vi "2D In Bounds Check.vi"(10 "Bounds":T2, 11 "Point in":cluster{"H":T1, "V":T1}) -> (2 "In Bounds?":bool, 3 "Point":cluster{"H":T1, "V":T1})   [LabVIEW 2022 SP3, in "FlexBlocks Support.lvlib"]
uses:
  FlexBlocks Support.lvlib
  <vilib>/XNodeSupport/XNodeInt.ctl
  <vilib>/XNodeSupport/NI_XNodeSupport.lvlib
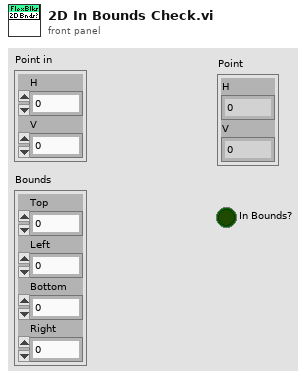
[diagram p1: front panel]
types:
  T1 = typedef "NI_XNodeSupport.lvlib/XNodeInt.ctl" = i32
  T2 = cluster{"Top":i32, "Left":i32, "Bottom":i32, "Right":i32}
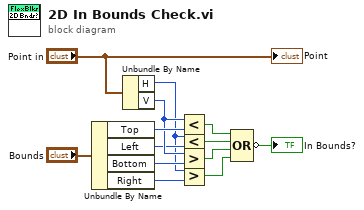
[diagram p0: block diagram]
diagram:
  n1 = Unbundle By Name("Bounds") -> ("Top"=w12:i32, "Left"=w9:i32, "Bottom"=w11:i32, "Right"=w8:i32)
  n2 = Unbundle By Name("Point in") -> ("H"=w2:T1, "V"=w10:T1)
  n3 = Less?(x=w10, y=w12) -> (x < y?=w6:bool)
  n4 = Less?(x=w2, y=w9) -> (x < y?=w7:bool)
  n5 = Greater?(x=w10, y=w11) -> (0:w5:bool)
  n6 = Greater?(x=w2, y=w8) -> (0:w4:bool)
  n7 = Compound Arithmetic op=OR(w6, w7, w5, w4) -> (invert →"In Bounds?":bool)
  "Point" <- "Point in"
